vi "alignTimes.vi"(8 "error in (no error)":errorcluster, 10 "sortedData":T2(array[cluster]), 11 "RfOutputData in":refnum<class "RfOutputData.lvclass">) -> (0 "error out":errorcluster, 2 "rfData":T1(array[cluster]) {"time" format="%_9g"}, 3 "RfOutputData out":refnum<class "RfOutputData.lvclass">)   [LabVIEW 2009, in "DataMappers.lvlib" / "RfOutputData.lvclass"]
uses:
  RfOutputData.lvclass
  DatabaseHelpers/Database Objects/Channel/RfOutputChannel/RfOutputChannel.lvclass
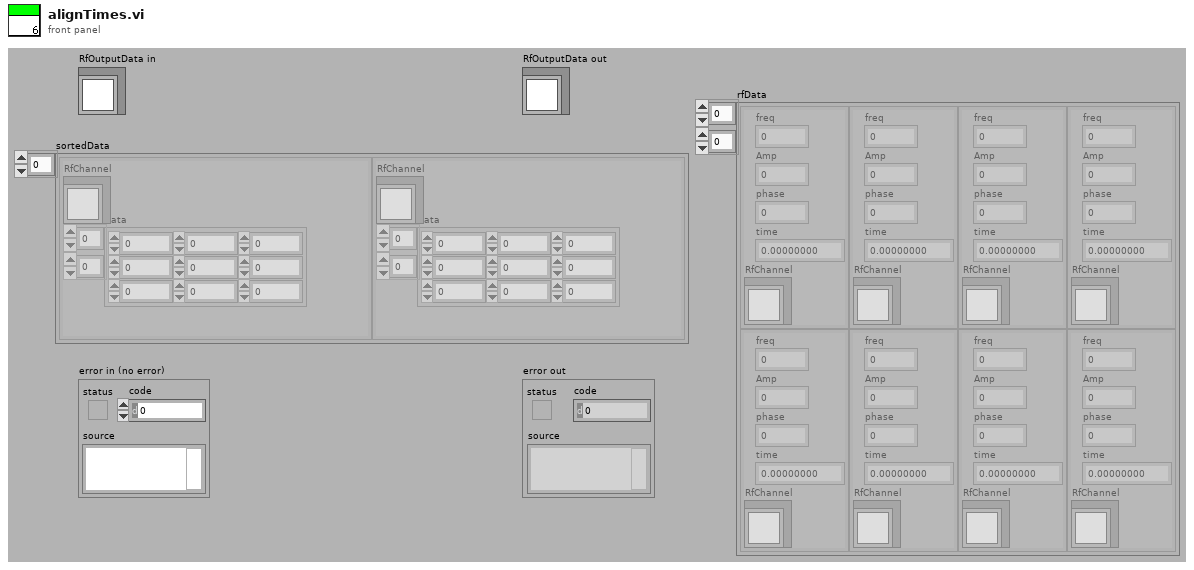
[diagram p1: front panel]
types:
  T1 = cluster{"freq":dbl, "Amp":dbl, "phase":dbl, "time":dbl, "RfChannel":refnum<class "RfOutputChannel.lvclass">}[][]
  T2 = cluster{"RfChannel":refnum<class "RfOutputChannel.lvclass">, "data":dbl[][]}[]
  T3 = cluster{"freq":dbl[], "Amp":dbl[], "phase":dbl[], "time":dbl[], "RfChannel":refnum<class "RfOutputChannel.lvclass">}
  T4 = cluster{"freq":dbl, "Amp":dbl, "phase":dbl, "time":dbl, "RfChannel":refnum<class "RfOutputChannel.lvclass">}
  T5 = cluster{"Frequency":dbl, "Amplitude":dbl, "Phase":dbl, "OutputForm":enum16{"Sine", "Square", "Triangle", "Arbitrary"}}
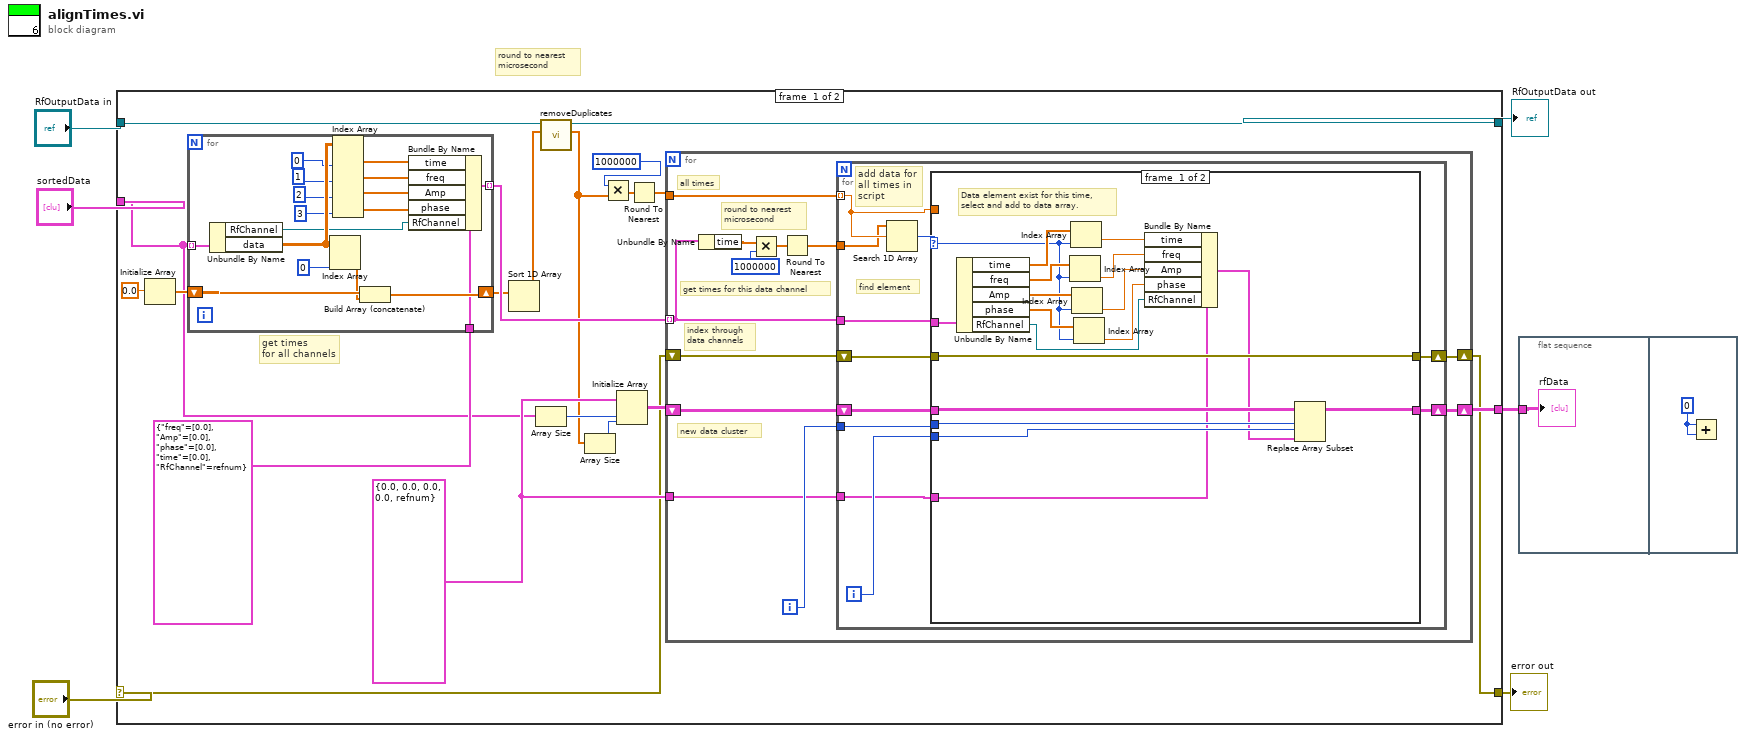
[diagram p0: block diagram]
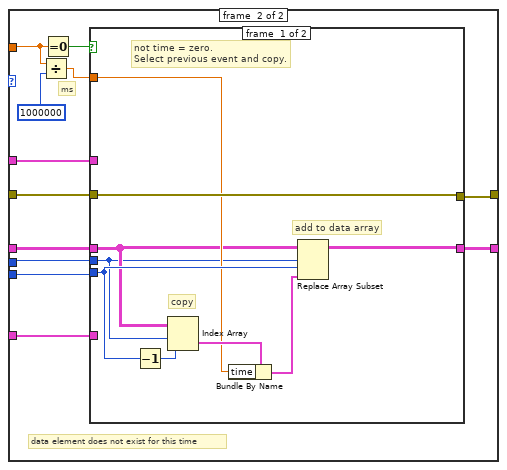
[diagram p2: hidden frame]
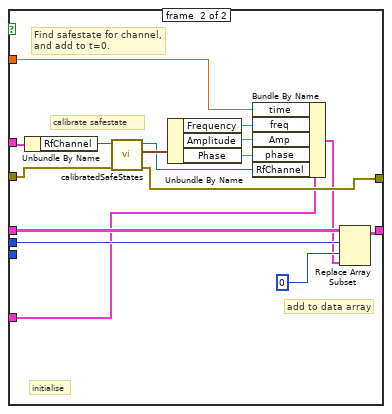
[diagram p3: hidden frame]
diagram:
  # "round to nearest\nmicrosecond"
  n1 = case shown="No Error" "error in (no error)" {
    selector: "error in (no error)" -> [w16 w123]
    tunnel: [w17 w123] -> w5
    tunnel: [w9 w122] -> w3
    tunnel: "RfOutputData in" -> [w11 w122]
    tunnel: "sortedData" -> [w15 _]
    tunnel: [w18 _] -> w1
    frame #0 {
      w21 = T4 {"freq"=0.0, "Amp"=0.0, "phase"=0.0, "time"=0.0, "RfChannel"=refnum}
      # "get times \nfor all channels"
      n2 = Initialize Array(0.0) -> (w25:dbl[])  [unwired: 1 in]
      n3 = for {
        tunnel: w15 -> [w121] mode=indexing
        shift-right: [w118] -> w13
        shift-left: w25 -> [w120]
        tunnel: T3 {"freq"=[0.0], "Amp"=[0.0], "phase"=[0.0], "time"=[0.0], "RfChannel"=refnum} -> [w112]
        tunnel: [w108] -> w22 mode=indexing
        n4 = Unbundle By Name(w121) -> ("RfChannel"=w105:refnum<class "RfOutputChannel.lvclass">, "data"=w117:dbl[][])
        n5 = Index Array(array=w117, index (col)=0) -> (element=w119:dbl[])  [unwired: 1 in]
        n6 = Index Array(array=w117, index (col) #1=0, index (col) #2=1, index (col) #3=2, index (col) #4=3) -> (element #1=w106:dbl[], element #2=w111:dbl[], element #3=w110:dbl[], element #4=w109:dbl[])  [unwired: 4 in]
        n7 = Build Array (concatenate)(w120, w119) -> (w118:dbl[])
        n8 = Bundle By Name(cluster=w112, "time"=w106, "freq"=w111, "Amp"=w110, "phase"=w109, "RfChannel"=w105) -> (w108:T3)
      }
      n9 = Sort 1D Array(array=w13) -> (sorted array=w10:dbl[])
      n10 = Array Size(array=w15) -> (size(s)=w14:i32)
      n11 = call "removeDuplicates.vi"("times"=w10, "RfOutputData in"=w11) -> ("times out"=w8:dbl[], "RfOutputData out"=w9:refnum<class "RfOutputData.lvclass">)  [unwired: 7 in, 1 out]
      n12 = Array Size(array=w8) -> (size(s)=w12:i32)
      n13 = Multiply(x=1000000, y=w8) -> (x*y=w20:dbl[])
      n14 = Initialize Array(w21, w14, w12) -> (w24:T1)
      n15 = Round To Nearest(number=w20) -> (nearest integer value=w19:dbl[])
      n16 = for {
        tunnel: w19 -> [w36]
        shift-right: [w38] -> w17
        shift-left: w16 -> [w37]
        tunnel: w22 -> [w29] mode=indexing
        shift-right: [w33] -> w18
        shift-left: w24 -> [w35]
        tunnel: w21 -> [w27]
        i -> [w34]
        # "new data cluster"
        # "all times"
        # "index through\ndata channels"
        # "get times for this data channel"
        # "round to nearest\nmicrosecond"
        n17 = Unbundle By Name(w29) -> ("time"=w28:dbl[])
        n18 = Multiply(x=w28, y=1000000) -> (x*y=w32:dbl[])
        n19 = Round To Nearest(number=w32) -> (nearest integer value=w30:dbl[])
        n20 = for {
          shift-right: [w47] -> w38
          shift-left: w37 -> [w48]
          tunnel: w36 -> [w45] mode=indexing
          shift-right: [w41] -> w33
          shift-left: w35 -> [w44]
          tunnel: w34 -> [w43]
          tunnel: w30 -> [w40]
          tunnel: w29 -> [w46]
          tunnel: w27 -> [w39]
          i -> [w42]
          # "add data for \nall times in\nscript"
          # "find element"
          n21 = Search 1D Array(1D array=w40, element=w45) -> (index of element=w49:i32)  [unwired: 1 in]
          n22 = case shown="-1" w49 {
            selector: w49 -> [w57 _]
            tunnel: w45 -> [_ w71]
            tunnel: w46 -> [w62 w78]
            tunnel: w48 -> [w67 w77]
            tunnel: [w67 w76] -> w47
            tunnel: w42 -> [w63 w75]
            tunnel: w44 -> [w66 w74]
            tunnel: w43 -> [w64 w73]
            tunnel: [w65 w72] -> w41
            tunnel: w39 -> [w56 w68]
            frame #0 {
              # "Data element exist for this time,\nselect and add to data array."
              n23 = Unbundle By Name(w62) -> ("time"=w61:dbl[], "freq"=w60:dbl[], "Amp"=w59:dbl[], "phase"=w58:dbl[], "RfChannel"=w51:refnum<class "RfOutputChannel.lvclass">)
              n24 = Index Array(array=w60, index=w57) -> (element=w54:dbl)
              n25 = Index Array(array=w61, index=w57) -> (element=w55:dbl)
              n26 = Index Array(array=w59, index=w57) -> (element=w53:dbl)
              n27 = Index Array(array=w58, index=w57) -> (element=w52:dbl)
              n28 = Bundle By Name(cluster=w56, "time"=w55, "freq"=w54, "Amp"=w53, "phase"=w52, "RfChannel"=w51) -> (w50:T4)
              n29 = Replace Array Subset(array=w66, new element=w50, index (row)=w64, index (col)=w63) -> (w65:T1)
            }
            frame #1 {
              # "ms"
              # "data element does not exist for this time"
              n30 = Divide(x=w71, y=1000000) -> (x/y=w70:dbl)
              n31 = Equal To 0?(x=w71) -> (x = 0?=w79:bool)
              n32 = case shown="True" w79 {
                tunnel: w70 -> [w84 w89]
                tunnel: w78 -> [_ w92]
                tunnel: w77 -> [w88 w99]
                tunnel: [w88 w98] -> w76
                tunnel: w75 -> [w86 _]
                tunnel: w74 -> [w82 w104]
                tunnel: w73 -> [w80 w101]
                tunnel: [w87 w103] -> w72
                tunnel: w68 -> [_ w91]
                frame #0 {
                  # "add to data array"
                  # "copy"
                  # "not time = zero.\nSelect previous event and copy."
                  n33 = Decrement(x=w86) -> (x-1=w81:i32)
                  n34 = Index Array(array=w82, index (row)=w80, index (col)=w81) -> (element=w85:T4)
                  n35 = Bundle By Name(cluster=w85, "time"=w84) -> (w83:T4)
                  n36 = Replace Array Subset(array=w82, new element=w83, index (row)=w80, index (col)=w86) -> (w87:T1)
                }
                frame #1 {
                  # "add to data array"
                  # "calibrate safestate"
                  # "Find safestate for channel,\nand add to t=0."
                  # "initialise"
                  n37 = Unbundle By Name(w92) -> ("RfChannel"=w100:refnum<class "RfOutputChannel.lvclass">)
                  n38 = call-dynamic "calibratedSafeStates.vi"("error in (no error)"=w99, "RfOutputChannel in"=w100) -> ("error out"=w98:errorcluster, "OutputDefaults"=w97:T5, "RfOutputChannel out"=w93:refnum<class "RfOutputChannel.lvclass">)  [unwired: 7 in]
                  n39 = Unbundle By Name(w97) -> ("Frequency"=w96:dbl, "Amplitude"=w95:dbl, "Phase"=w94:dbl)
                  n40 = Bundle By Name(cluster=w91, "time"=w89, "freq"=w96, "Amp"=w95, "phase"=w94, "RfChannel"=w93) -> (w90:T4)
                  n41 = Replace Array Subset(array=w104, new element=w90, index (row)=w101, index (col)=0) -> (w103:T1)
                }
              }
            }
          }
        }
      }
    }
    frame #1 {
    }
  }
  "error out" <- w5
  "RfOutputData out" <- w3
  n42 = flat-sequence {
    tunnel: w1 -> [w124]
    frame #0 {
      "rfData" <- w124
    }
    frame #1 {
      w125 = 0
      n43 = Add(x=w125, y=w125) -> ()  [unwired: 1 out]
    }
  }
